vi "ExOpenSpectTestGlobal.vi"() -> ()   [LabVIEW 2010]
uses:
  GlbCamHndls.vi
panel:
  out "Total number of Spectrometers defined in system":u32
  out "Array":bool[](array[boolean])
  out "Total Spectrometer array size":u32
  out "error out":errorcluster
  in  "error in (no error)":errorcluster
  in  "Spectrometer Number to open":u32=1 min=1 step=1
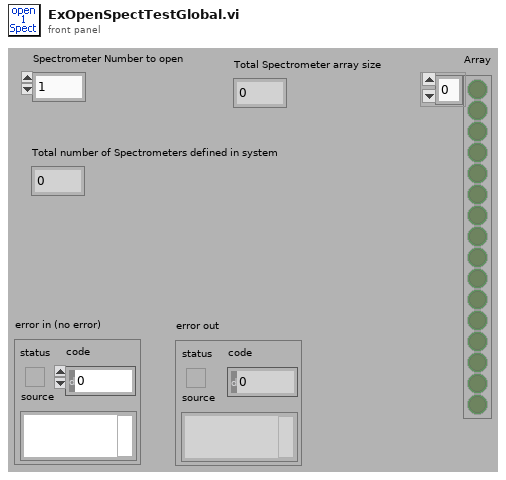
[diagram p1: front panel]
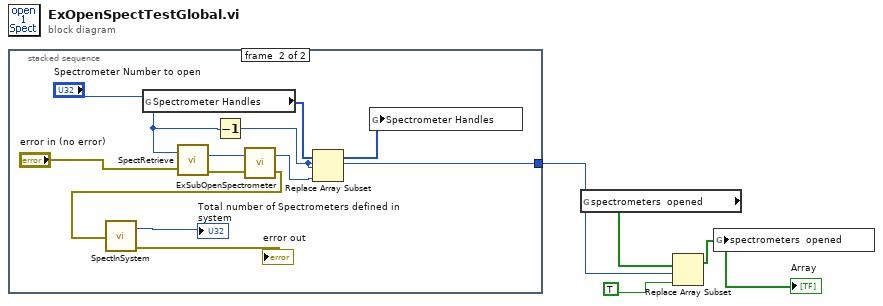
[diagram p0: block diagram]
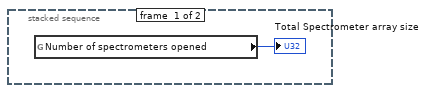
[diagram p2: hidden frame]
diagram:
  n1 = stacked-sequence {
    tunnel: [_ w10] -> w4
    frame #0 {
      n2 = global read "GlbCamHndls.vi" "Number of spectrometers opened"() -> (→"Total Spectrometer array size":u32)
    }
    frame #1 {
      n3 = global read "GlbCamHndls.vi" "Spectrometer Handles"() -> (w14:u32[])
      n4 = call <userlib>:"SpectRetrieve.vi"("error in"="error in (no error)", "Index"="Spectrometer Number to open") -> ("error out"=w16:errorcluster, "Device ID"=w15:u32)
      n5 = Decrement(x="Spectrometer Number to open") -> (x-1=w10:u32)
      n6 = call "ExSubOpenSpectrometer.vi"("error in (no error)"=w16, "Spectrometer Device ID"=w15) -> ("error out"=w6:errorcluster, "Spectrometer Handle"=w13:u32)
      n7 = call <userlib>:"SpectInSystem.vi"("error in"=w6) -> ("Number of Spectrographs"=→"Total number of Spectrometers defined in system":i32, "error out"=→"error out":errorcluster)
      n8 = Replace Array Subset(array=w14, new element=w13, index=w10) -> (w11:u32[])
      n9 = global write "GlbCamHndls.vi" "Spectrometer Handles"(w11) -> ()
    }
  }
  n10 = global read "GlbCamHndls.vi" "spectrometers  opened"() -> (w2:bool[])
  n11 = Replace Array Subset(array=w2, new element=TRUE, index=w4) -> (w1:bool[])
  "Array" <- w1
  n12 = global write "GlbCamHndls.vi" "spectrometers  opened"(w1) -> ()
